vi "Parse Error XML.vi"(9 "Code Tag Value":string, 10 "Error XML":string, 11 "AWS Core":refnum<class "Bucket.lvclass">) -> (1 "Error Description Override":string, 2 "Error Code":i32, 3 "Warning":bool)   [LabVIEW 2015, in "NI_AWS_S3.lvlib" / "Bucket.lvclass"]
uses:
  Bucket.lvclass
  Core/HTTP Request/HTTP Request.lvclass
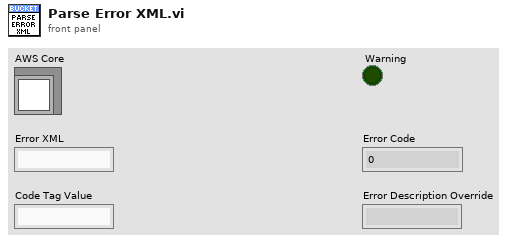
[diagram p1: front panel]
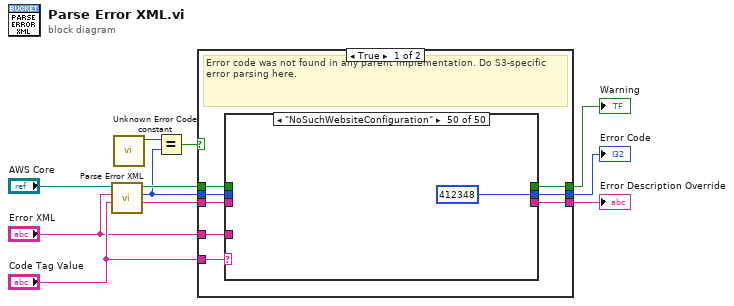
[diagram p0: block diagram]
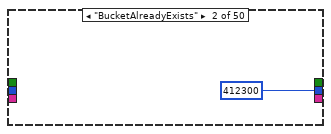
[diagram p3: hidden frame]
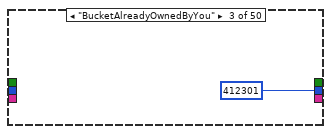
[diagram p4: hidden frame]
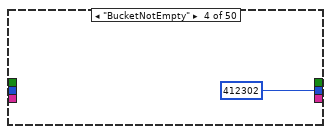
[diagram p5: hidden frame]
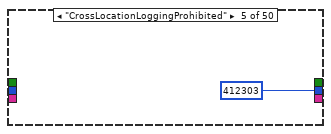
[diagram p6: hidden frame]
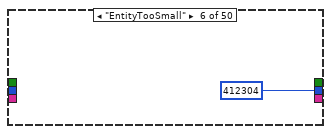
[diagram p7: hidden frame]
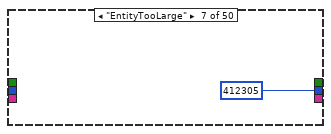
[diagram p8: hidden frame]
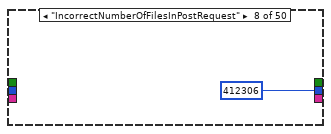
[diagram p9: hidden frame]
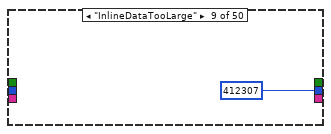
[diagram p10: hidden frame]
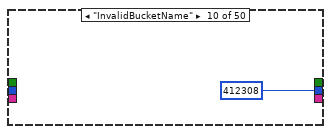
[diagram p11: hidden frame]
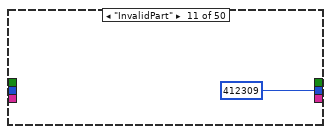
[diagram p12: hidden frame]
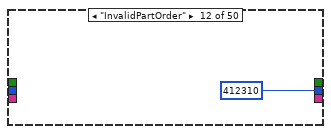
[diagram p13: hidden frame]
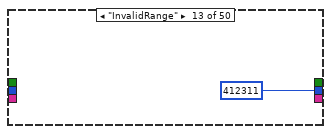
[diagram p14: hidden frame]
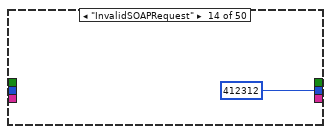
[diagram p15: hidden frame]
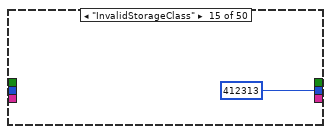
[diagram p16: hidden frame]
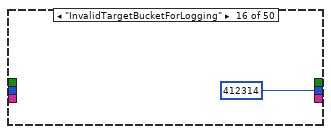
[diagram p17: hidden frame]
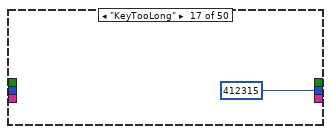
[diagram p18: hidden frame]
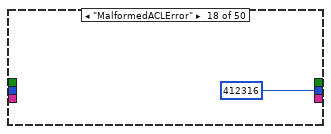
[diagram p19: hidden frame]
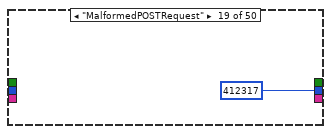
[diagram p20: hidden frame]
diagram:
  n1 = call-parent "Parse Error XML.vi"("Code Tag Value"="Code Tag Value", "Error XML"="Error XML", "AWS Core"="AWS Core") -> ("Error Description Override"=w7:string, "Error Code"=w1:i32, "Warning"=w8:bool)  [unwired: 6 in]
  n2 = call "Unknown Error Code constant.vi"() -> ("AWS Unknown Error Code value"=w10:i32)  [unwired: 11 in]
  n3 = Equal?(x=w10, y=w1) -> (x = y?=w9:bool)
  n4 = case shown="True" w9 {
    tunnel: w8 -> [w17 w74]
    tunnel: w7 -> [w15 w73]
    tunnel: [w14 w74] -> w2
    tunnel: [w12 w73] -> w4
    tunnel: [w13 w72] -> w3
    tunnel: "Error XML" -> [w18 _]
    tunnel: "Code Tag Value" -> [w19 _]
    tunnel: w1 -> [w16 w72]
    frame True {
      # "Error code was not found in any parent implementation. Do S3-specific error parsing here."
      n5 = case shown="\"NoSuchWebsiteConfiguration\"" w19 {
        tunnel: [w21 412300 412301 412302 412303 412304 412305 412306 412307 412308 412309 412310 412311 412312 412313 412314 412315 412316 412317 412318 412319 412320 412321 412322 412323 412324 412325 412326 412327 412328 412329 412330 412331 412332 412333 412334 412335 412336 412337 412338 412339 412340 412341 412342 412343 412344 412345 412346 412347 412348] -> w13
        tunnel: w18 -> [_ _ _ _ _ _ _ _ _ _ _ _ _ _ _ _ _ _ _ _ _ _ _ _ _ _ _ _ _ _ _ _ _ _ _ _ _ _ _ _ _ _ _ _ _ _ _ _ _ _]
        tunnel: w17 -> [w22 _ _ _ _ _ _ _ _ _ _ _ _ _ _ _ _ _ _ _ _ _ _ _ _ _ _ _ _ _ _ _ _ _ _ _ _ _ _ _ _ _ _ _ _ _ _ _ _ _]
        tunnel: w16 -> [w21 _ _ _ _ _ _ _ _ _ _ _ _ _ _ _ _ _ _ _ _ _ _ _ _ _ _ _ _ _ _ _ _ _ _ _ _ _ _ _ _ _ _ _ _ _ _ _ _ _]
        tunnel: w15 -> [w20 _ _ _ _ _ _ _ _ _ _ _ _ _ _ _ _ _ _ _ _ _ _ _ _ _ _ _ _ _ _ _ _ _ _ _ _ _ _ _ _ _ _ _ _ _ _ _ _ _]
        tunnel: [w22 _ _ _ _ _ _ _ _ _ _ _ _ _ _ _ _ _ _ _ _ _ _ _ _ _ _ _ _ _ _ _ _ _ _ _ _ _ _ _ _ _ _ _ _ _ _ _ _ _] -> w14
        tunnel: [w20 _ _ _ _ _ _ _ _ _ _ _ _ _ _ _ _ _ _ _ _ _ _ _ _ _ _ _ _ _ _ _ _ _ _ _ _ _ _ _ _ _ _ _ _ _ _ _ _ _] -> w12
        frame Default {
          # "Unknown error code, use default error from parent"
        }
        frame "BucketAlreadyExists" {
        }
        frame "BucketAlreadyOwnedByYou" {
        }
        frame "BucketNotEmpty" {
        }
        frame "CrossLocationLoggingProhibited" {
        }
        frame "EntityTooSmall" {
        }
        frame "EntityTooLarge" {
        }
        frame "IncorrectNumberOfFilesInPostRequest" {
        }
        frame "InlineDataTooLarge" {
        }
        frame "InvalidBucketName" {
        }
        frame "InvalidPart" {
        }
        frame "InvalidPartOrder" {
        }
        frame "InvalidRange" {
        }
        frame "InvalidSOAPRequest" {
        }
        frame "InvalidStorageClass" {
        }
        frame "InvalidTargetBucketForLogging" {
        }
        frame "KeyTooLong" {
        }
        frame "MalformedACLError" {
        }
        frame "MalformedPOSTRequest" {
        }
        frame "MaxMessageLengthExceeded" {
        }
        frame "MaxPostPreDataLengthExceededError" {
        }
        frame "MetadataTooLarge" {
        }
        frame "MissingAttachment" {
        }
        frame "MissingContentLength" {
        }
        frame "MissingRequestBodyError" {
        }
        frame "MissingSecurityElement" {
        }
        frame "MissingSecurityHeader" {
        }
        frame "NoLoggingStatusForKey" {
        }
        frame "NoSuchBucket" {
        }
        frame "NoSuchKey" {
        }
        frame "NoSuchUpload" {
        }
        frame "NotSignedUp" {
        }
        frame "OperationAborted" {
        }
        frame "PermanentRedirect" {
        }
        frame "RequestIsNotMultiPartContent" {
        }
        frame "RequestTorrentOfBucketError" {
        }
        frame "TokenRefreshRequired" {
        }
        frame "TooManyBuckets" {
        }
        frame "UnexpectedContent" {
        }
        frame "UnresolvableGrantByEmailAddress" {
        }
        frame "UserKeyMustBeSpecified" {
        }
        frame "NoSuchBucketPolicy" {
        }
        frame "InvalidBucketState" {
        }
        frame "InvalidEncryptionAlgorithmError" {
        }
        frame "InvalidObjectState" {
        }
        frame "InvalidRequest" {
        }
        frame "NoSuchLifecycleConfiguration" {
        }
        frame "RestoreAlreadyInProgress" {
        }
        frame "ServiceUnavailable" {
        }
        frame "NoSuchWebsiteConfiguration" {
        }
      }
    }
    frame False {
      # "Parent method already assigned an error code"
    }
  }
  "Error Description Override" <- w4
  "Warning" <- w2
  "Error Code" <- w3
